vi "AFT Filter Signal (Complex, PtByPt).vi"(7 "reset? (F)":bool, 8 "error in (no error)":errorcluster, 10 "x(n)":cdb, 11 "adaptive filter in":refnum<k20>) -> (0 "error out":errorcluster, 2 "y(n)":cdb, 3 "adaptive filter out":refnum<k20>)   [LabVIEW 2017, in "NI_AdaptiveFilter.lvlib"]
doc: "Filters an input signal with an adaptive filter point by point. You must use the least mean squares (LMS) or recursive least squares (RLS) algorithms to create the adaptive filter. Unlike the AFT Filter Signal and Update Coefficients VI, the AFT Filter Signal VI does not update the coefficients of the adaptive filter. Use the AFT Update Coefficients VI to update the filter coefficients. Wire data to the <B>x(n)</B> input to determine the polymorphic instance to use or manually select the instance. The data type of the adaptive filter that you wire to the <B>adaptive filter in</B> input must match the instance of the AFT Filter Signal VI."
uses:
  <vilib>/addons/Adaptive Filters/NI_AdaptiveFilter.lvlib
  <resource>/AdaptiveFilters.dll
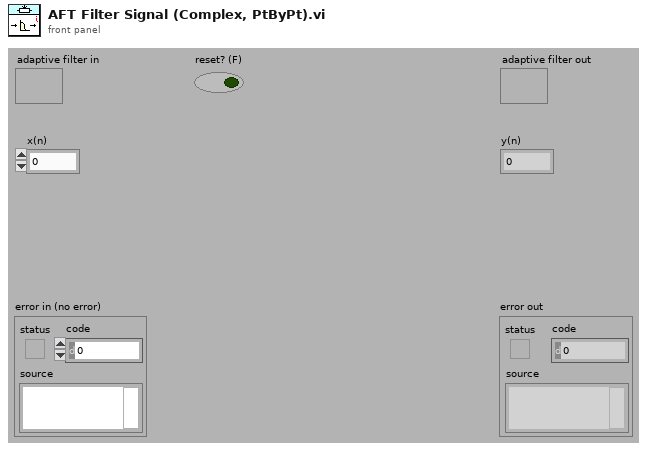
[diagram p1: front panel]
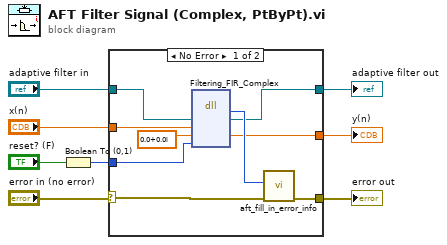
[diagram p0: block diagram]
diagram:
  n1 = Boolean To (0,1)(Boolean="reset? (F)") -> (0, 1=w5:i16)
  n2 = case shown="No Error" "error in (no error)" {
    selector: "error in (no error)" -> [w16 w19]
    tunnel: [w14 w19] -> w8
    tunnel: "adaptive filter in" -> [w10 w18]
    tunnel: "x(n)" -> [w17 _]
    tunnel: [w9 w18] -> w2
    tunnel: w5 -> [w13 _]
    tunnel: [w12 _] -> w1
    frame No Error {
      n3 = dll-call lib="C:/Program Files/National Instruments/LabVIEW 2017/resource/AdaptiveFilters.dll" fn="Filtering_FIR_Complex" ("Complex Data Initialization")("pSession"=w10, "x"=w17, "y"=cdb 0.0+0.0i ("y(n) 2"), "reset"=w13) -> ("err"=w15:i32, "pSession"=w9:refnum<k20>, "y"=w12:cdb)  [unwired: 5 in, 2 out]
      n4 = call <vilib>:"aft_fill_in_error_info.vi"("error in"=w16, "status code"=w15) -> ("error out"=w14:errorcluster)  [unwired: 2 in, 7 out]
    }
    frame Error {
    }
  }
  "error out" <- w8
  "y(n)" <- w1
  "adaptive filter out" <- w2
